vi "Host Run Resolver Sim.vi"() -> ()   [LabVIEW 2010]
uses:
  <vilib>/rvi/interface/nirviCloseFPGA/nirviCloseFPGA.xnode
  <vilib>/rvi/interface/nirviOpenFPGA/nirviOpenFPGA.xnode
  <vilib>/userDefined/High Color/nirio_resource_hc.ctl
  <vilib>/rvi/interface/nirviReadWriteControl/nirviReadWriteControl.xnode
  FPGA/FPGA 5 Wire xVDT Sim.vi
  FPGA Bitfiles/ResolverSimulati_7852_FPGA5WirexVDTSim_D77CF6EF.lvbitx
  <vilib>/RVI Host/nirviSupport.llb/nirviErrorClusterFromErrorCode.vi
  <vilib>/rvi/errors/niLvFpgaWhatHappensToTopLevelVI.ctl
  <vilib>/rvi/interface/common/niFpgaNodeNameForErrorReporting.ctl
  <vilib>/rvi/errors/niLvFpgaAdjustHostInterfaceError.vi
  <vilib>/FPGAPlugInAG/PXI-7852R/niLvFpga_Close_PXI-7852R.vi
panel:
  out "Scaling Factor 2":fxp<+/-,19,5> format="%.16g"
  out "Scaling Factor":fxp<+/-,19,5> format="%.16g"
  out "error out":errorcluster
  in  "stop":bool
  in  "Position (deg)":dbl(slide) caption="Position" scale=0.0..360.0 scale format="%.2f"
  # "Run-Time"
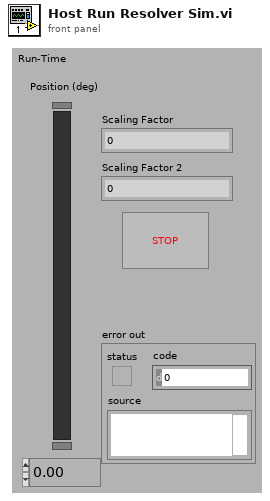
[diagram p1: front panel]
types:
  T1 = typedef "niFpgaNodeNameForErrorReporting.ctl" = enum16{"Open FPGA VI Reference", "Read/Write Control", "Invoke Method: Abort", "Invoke Method: Acknowledge IRQ", "Invoke Method: Download", "Invoke Method: FIFO.Configure", "Invoke Method: FIFO.Read", "Invoke Method: FIFO.Start", "Invoke Method: FIFO.Stop", "Invoke Method: FIFO.Write", "Invoke Method: Reset", "Invoke Method: Run", "Invoke Method: Wait on IRQ", "Close FPGA VI Reference"}
  T2 = typedef "niLvFpgaWhatHappensToTopLevelVI.ctl" = enum16{"top level VI scripted behind XNode", "top level VI inlined behind XNode"}
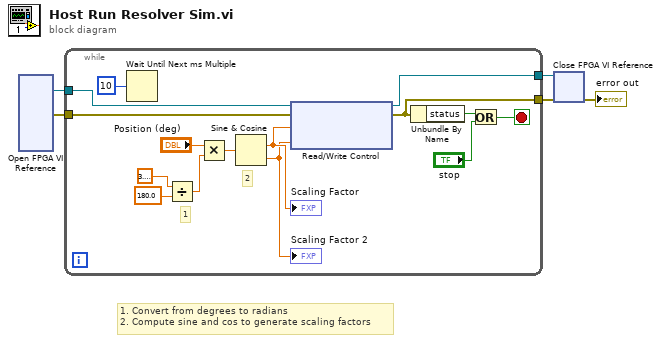
[diagram p0: block diagram]
diagram:
  # "1. Convert from degrees to radians\n2. Compute sine and cos to generate scaling factors"
  n1 = xnode "Open FPGA VI Reference"() -> ("FPGA VI Reference Out"=w3:refnum<k20>, "error out"=w2:errorcluster)  [unwired: 2 in]
  n2 = while {
    tunnel: w2 -> [w14]
    tunnel: [w16] -> w5
    tunnel: w3 -> [w15]
    tunnel: [w13] -> w1
    stop <- w18 stop-if-true
    # "2"
    # "1"
    n3 = Wait Until Next ms Multiple(millisecond multiple=u32 10) -> ()  [unwired: 1 out]
    n4 = Divide(x=3.141592653589793, y=180.0) -> (x/y=w10:dbl)
    n5 = Multiply(x="Position (deg)", y=w10) -> (x*y=w9:dbl)
    n6 = Sine & Cosine(0:w9) -> (1:w7:dbl, 2:w6:dbl)
    "Scaling Factor" <- w7
    "Scaling Factor 2" <- w6
    n7 = xnode "Read/Write Control"("FPGA VI Reference In"=w15, "error in"=w14, "Scaling Factor"=w7, "Scaling Factor 2"=w6) -> ("FPGA VI Reference Out"=w13:refnum<k20>, "error out"=w16:errorcluster)
    n8 = Unbundle By Name(w16) -> ("status"=w17:bool)
    n9 = Or(x=w17, y="stop") -> (x .or. y?=w18:bool)
  }
  n10 = xnode "Close FPGA VI Reference"("FPGA VI Reference In"=w1, "error in"=w5) -> ("error out"=→"error out":errorcluster)
